vi "GetValue.vi"(8 "error in":errorcluster, 11 "DateTimeMeasure in":refnum<class "DateTimeMeasure.lvclass">) -> (0 "error out":errorcluster, 2 "Value":timestamp, 3 "DateTimeMeasure out":refnum<class "DateTimeMeasure.lvclass">)   [LabVIEW 2021, in "ProligentXMLGenerator.lvlib" / "DateTimeMeasure.lvclass"]
doc: "Defines the value acquired by the measure."
uses:
  DateTimeMeasure.lvclass
  DateTimeMeasure.lvclass/DateTimeMeasure.ctl
  Base/DateTime/DateTime.lvclass
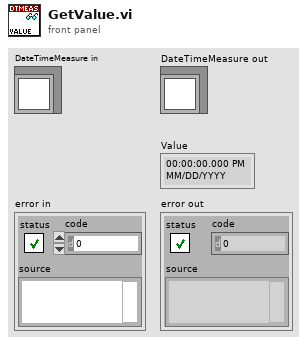
[diagram p1: front panel]
types:
  T1 = typedef "ProligentXMLGenerator.lvlib/DateTimeMeasure.lvclass/Data.ctl" = cluster{"Value":refnum<class "DateTime.lvclass">, "TimeZoneInfoId":string}
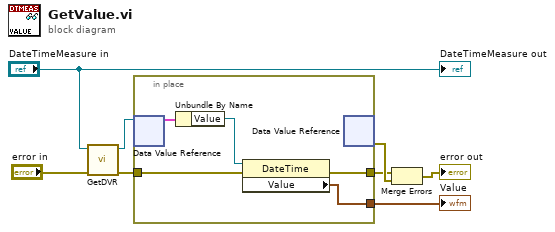
[diagram p0: block diagram]
diagram:
  n1 = call "GetDVR.vi"("error in"="error in", "DateTimeMeasure"="DateTimeMeasure in") -> ("error out"=w2:errorcluster, "DVRReference"=w7:refnum<data-value>)  [unwired: 8 in]
  n2 = in-place "In Place Element Structure" {
    in-place-border: [w9] -> w6
    in-place-border: w2 -> [w11]
    in-place-border: [w10] -> w1
    n3 = in-place-dvr #1(w7) -> (w13:T1)  [unwired: 1 out]
    n4 = Unbundle By Name(w13) -> ("Value"=w12:refnum<class "DateTime.lvclass">)
    n5 = property class="DateTime"(reference=w12, error in=w11) -> (error out=w10:errorcluster, "Value"=w9:timestamp)  [unwired: 1 out]
    n6 = in-place-dvr #1() -> (w8:errorcluster)  [unwired: 1 in, 1 out]
  }
  "Value" <- w6
  n7 = Merge Errors(w1, w8) -> (→"error out":errorcluster)
  "DateTimeMeasure out" <- "DateTimeMeasure in"
